vi "UPRcontroller_v00_basedonlsmv66.vi"() -> ()   [LabVIEW 2015] (continued)
                    n2964 = local read "square matrix"() -> (w6486:bool)
                    n2965 = local read "Vx-max ref"() -> (w6492:dbl)
                    n2966 = local read "Vx-min ref"() -> (w6491:dbl)
                    n2967 = local read "Vy-min ref"() -> (w6488:dbl)
                    n2968 = local read "ypixels ref"() -> (w6490:i32)
                    n2969 = local read "Vy-max ref"() -> (w6489:dbl)
                    n2970 = local read "xpixels ref"() -> (w6493:i32)
                    n2971 = local read "Angle ref"() -> (w6485:dbl)
                    n2972 = local read "Colormap"() -> (w6494:i32)
                    n2973 = call "2pparameters.vi"("command"="get") -> ("params out"=w6497:T12)  [unwired: 1 in]
                    n2974 = Bundle By Name(cluster=w6497, "Xpixels Img"=w6493, "Vx-min Img"=w6491, "VX-max Img"=w6492, "Ypixels Img"=w6490, "Vy-min Img"=w6488, "Vy-max Img"=w6489, "Colormap"=w6494, "square pixels"=w6487, "square matrix"=w6486, "Angle Img"=w6485) -> (w6496:T12)
                    n2975 = call "2pparameters.vi"("Params in"=w6496, "command"="set") -> ()  [unwired: 1 out]
                    n2976 = local read "Vx-max draw"() -> (w6477:dbl)
                    n2977 = local read "Angle drawing"() -> (w6484:dbl)
                    n2978 = local read "Vx-min draw"() -> (w6478:dbl)
                    n2979 = local read "Vy-min draw"() -> (w6481:dbl)
                    n2980 = local read "ypixels draw"() -> (w6479:dbl)
                    n2981 = local read "Vy-max draw"() -> (w6480:dbl)
                    n2982 = local read "Square pixels"() -> (w6482:bool)
                    n2983 = local read "square matrix"() -> (w6483:bool)
                    n2984 = local read "xpixels draw"() -> (w6476:dbl)
                    n2985 = local read "Colormap"() -> (w6475:i32)
                    n2986 = call "2pparameters.vi"("command"="get") -> ("params out"=w6472:T12)  [unwired: 1 in]
                    n2987 = Bundle By Name(cluster=w6472, "Xpixels"=w6476, "Vxminref"=w6478, "Vxmaxref"=w6477, "Ypixels"=w6479, "Vyminref"=w6481, "Vymaxref"=w6480, "Colormap"=w6475, "square pixels"=w6482, "square matrix"=w6483, "Angle draw"=w6484) -> (w6473:T12)
                    n2988 = call "2pparameters.vi"("Params in"=w6473, "command"="set") -> ()  [unwired: 1 out]
                  }
                  frame #1 {
                    n2989 = Current VI's Path() -> (path=w6508:path)
                    n2990 = Strip Path(path=w6508) -> (stripped path=w6509:path)  [unwired: 1 out]
                    n2991 = Build Path(base path=w6509, name or relative path="subVIs\\Image\\SetROI_v4.vi") -> (appended path=w6507:path)
                    n2992 = call <vilib>:"Set Busy.vi"() -> ("error out"=w6505:errorcluster)  [unwired: 10 in, 1 out]
                    n2993 = Open VI Reference(type specifier VI Refnum (for type only)=refnum<vi> refnum, vi path=w6507, error in (no error)=w6505) -> (vi reference=w6503:refnum<vi>, error out=w6501:errorcluster)  [unwired: 3 in]
                    n2994 = call-by-ref "?"(reference=w6503, error in=w6501) -> (reference out=w6502:refnum<vi>, error out=w6500:errorcluster)  [unwired: 1 in]
                    n2995 = Close Reference(reference=w6502, error in (no error)=w6500) -> (error out=w6504:errorcluster)
                    n2996 = call <vilib>:"Unset Busy.vi"("error in (no error)"=w6504) -> ()  [unwired: 10 in, 1 out]
                    n2997 = local write "status"(w6504) -> ()
                  }
                  frame #2 {
                    n2998 = call "2pparameters.vi"("command"="get") -> ("params out"=w6534:T12)  [unwired: 1 in]
                    n2999 = Unbundle By Name(w6534) -> ("Xpixels Img"=w6533:i32, "Vx-min Img"=w6532:dbl, "VX-max Img"=w6531:dbl, "Ypixels Img"=w6530:i32, "Vy-min Img"=w6529:dbl, "Vy-max Img"=w6528:dbl, "Colormap"=w6527:u16, "square pixels"=w6526:bool, "square matrix"=w6525:bool, "Angle Img"=w6524:dbl, "Drawing Mode"=w6523:u16)
                    n3000 = local write "xpixels ref"(w6533) -> ()
                    n3001 = local write "Vx-min ref"(w6532) -> ()
                    n3002 = local write "Vx-max ref"(w6531) -> ()
                    n3003 = local write "ypixels ref"(w6530) -> ()
                    n3004 = local write "Vy-min ref"(w6529) -> ()
                    n3005 = local write "Vy-max ref"(w6528) -> ()
                    n3006 = local write "Colormap"(w6527) -> ()
                    n3007 = local write "Square pixels"(w6526) -> ()
                    n3008 = local write "square matrix"(w6525) -> ()
                    n3009 = local write "Angle ref"(w6524) -> ()
                    n3010 = local write "ROI Type"(w6523) -> ()
                    n3011 = call "2pparameters.vi"("command"="get") -> ("params out"=w6517:T12)  [unwired: 1 in]
                    n3012 = Unbundle By Name(w6517) -> ("Xpixels"=w6511:i32, "Vxminref"=w6515:dbl, "Vxmaxref"=w6514:dbl, "Ypixels"=w6510:i32, "Vyminref"=w6513:dbl, "Vymaxref"=w6512:dbl, "Colormap"=w6518:u16, "square pixels"=w6519:bool, "square matrix"=w6520:bool, "Angle draw"=w6521:dbl, "Drawing Mode"=w6522:u16)
                    n3013 = local write "Vy-max draw"(w6512) -> ()
                    n3014 = local write "Angle drawing"(w6521) -> ()
                    n3015 = local write "Colormap"(w6518) -> ()
                    n3016 = local write "Square pixels"(w6519) -> ()
                    n3017 = local write "square matrix"(w6520) -> ()
                    n3018 = local write "ROI Type"(w6522) -> ()
                    n3019 = local write "xpixels draw"(w6511) -> ()
                    n3020 = local write "ypixels draw"(w6510) -> ()
                    n3021 = local write "Vx-min draw"(w6515) -> ()
                    n3022 = local write "Vx-max draw"(w6514) -> ()
                    n3023 = local write "Vy-min draw"(w6513) -> ()
                  }
                  frame #3 {
                    n3024 = property on="ROI" class="Bool (strict)"("Val(Sgnl)"=FALSE ("x/y scan")) -> ()  [unwired: 2 in, 2 out]
                  }
                }
              }
            }
          }
          event "Xdattype": Value Change {
            n3025 = event-data() -> ()  [unwired: 1 in, 1 out]
            n3026 = case shown="True" "Xdattype" {
              frame False {
              }
              frame True {
                n3027 = stacked-sequence {
                  frame #0 {
                    n3028 = Current VI's Path() -> (path=w6547:path)
                    n3029 = Strip Path(path=w6547) -> (stripped path=w6548:path)  [unwired: 1 out]
                    n3030 = Build Path(base path=w6548, name or relative path="subVIs\\Misc\\Changedataconfig.vi") -> (appended path=w6546:path)
                    n3031 = call <vilib>:"Set Busy.vi"() -> ("error out"=w6544:errorcluster)  [unwired: 10 in, 1 out]
                    n3032 = Open VI Reference(type specifier VI Refnum (for type only)=refnum<vi> refnum, vi path=w6546, error in (no error)=w6544) -> (vi reference=w6539:refnum<vi>, error out=w6541:errorcluster)  [unwired: 3 in]
                    n3033 = call-by-ref "?"(reference=w6539, error in=w6541) -> (reference out=w6543:refnum<vi>, error out=w6542:errorcluster)  [unwired: 12 in]
                    n3034 = Close Reference(reference=w6543, error in (no error)=w6542) -> (error out=w6538:errorcluster)
                    "status" <- w6538
                    n3035 = call <vilib>:"Unset Busy.vi"("error in (no error)"=w6538) -> ()  [unwired: 10 in, 1 out]
                  }
                  frame #1 {
                    n3036 = property on="Xdattype" class="Bool (strict)"("Val(Sgnl)"=FALSE ("x/y scan")) -> ()  [unwired: 2 in, 2 out]
                  }
                }
              }
            }
          }
          event "XautoOD": Value Change {
            n3037 = event-data() -> ()  [unwired: 1 in, 1 out]
            n3038 = case shown="True" "XautoOD" {
              frame False {
              }
              frame True {
                n3039 = stacked-sequence {
                  frame #0 {
                    n3040 = Current VI's Path() -> (path=w6560:path)
                    n3041 = Strip Path(path=w6560) -> (stripped path=w6561:path)  [unwired: 1 out]
                    n3042 = Build Path(base path=w6561, name or relative path="subVIs\\Misc\\ChangeautoODs.vi") -> (appended path=w6559:path)
                    n3043 = call <vilib>:"Set Busy.vi"() -> ("error out"=w6557:errorcluster)  [unwired: 10 in, 1 out]
                    n3044 = Open VI Reference(type specifier VI Refnum (for type only)=refnum<vi> refnum, vi path=w6559, error in (no error)=w6557) -> (vi reference=w6552:refnum<vi>, error out=w6554:errorcluster)  [unwired: 3 in]
                    n3045 = call-by-ref "?"(reference=w6552, error in=w6554) -> (reference out=w6556:refnum<vi>, error out=w6555:errorcluster)  [unwired: 12 in]
                    n3046 = Close Reference(reference=w6556, error in (no error)=w6555) -> (error out=w6551:errorcluster)
                    "status 2" <- w6551
                    n3047 = call <vilib>:"Unset Busy.vi"("error in (no error)"=w6551) -> ()  [unwired: 10 in, 1 out]
                  }
                  frame #1 {
                    n3048 = property on="XautoOD" class="Bool (strict)"("Val(Sgnl)"=FALSE ("x/y scan")) -> ()  [unwired: 2 in, 2 out]
                  }
                }
              }
            }
          }
          event "SetMan": Value Change {
            n3049 = event-data() -> ()  [unwired: 1 in, 1 out]
            n3050 = case shown="True" "SetMan" {
              frame False {
              }
              frame True {
                n3051 = stacked-sequence {
                  frame #0 {
                    w6564 = u16 0 items=["Rectangle", "Circle", "Freeform Boundary", "Freeform Interior"] ("ROI Type")
                    n3052 = local write "ROI Type"(w6564) -> ()
                    n3053 = local read "Square pixels"() -> (w6570:bool)
                    n3054 = case shown="False" w6570 {
                      frame False {
                        n3055 = local read "square matrix"() -> (w6571:bool)
                        n3056 = case shown="False" w6571 {
                          frame False {
                            "ypixels ref" <- "ypixels"
                            "xpixels ref" <- "xpixels"
                          }
                          frame True {
                            n3057 = local read "xpixels"() -> (w6576:i32)
                            n3058 = local read "ypixels"() -> (w6575:i32)
                            n3059 = Max & Min(x=w6576, y=w6575) -> (max(x,y)=w6574:i32)  [unwired: 1 out]
                            n3060 = local write "xpixels ref"(w6574) -> ()
                            n3061 = local write "ypixels ref"(w6574) -> ()
                          }
                        }
                      }
                      frame True {
                        n3062 = local read "square matrix"() -> (w6577:bool)
                        n3063 = case shown="True" w6577 {
                          frame False {
                            n3064 = local read "Vxmax"() -> (w6591:dbl)
                            n3065 = local read "Vx-min"() -> (w6590:dbl)
                            n3066 = local read "Vy-max"() -> (w6586:dbl)
                            n3067 = local read "Vy-min"() -> (w6587:dbl)
                            n3068 = Subtract(x=w6586, y=w6587) -> (x-y=w6588:dbl)
                            n3069 = Subtract(x=w6591, y=w6590) -> (x-y=w6589:dbl)
                            n3070 = Absolute Value(x=w6588) -> (abs(x)=w6579:dbl)
                            n3071 = Absolute Value(x=w6589) -> (abs(x)=w6580:dbl)
                            n3072 = Divide(x=w6580, y=w6579) -> (x/y=w6585:dbl)
                            n3073 = Greater Or Equal?(x=w6580, y=w6579) -> (x >= y?=w6578:bool)
                            n3074 = local read "xpixels"() -> (w6584:i32)
                            n3075 = local read "ypixels"() -> (w6581:i32)
                            n3076 = case shown="False" w6578 {
                              tunnel: w6585 -> [w6596 w6599]
                              tunnel: w6584 -> [w6593 _]
                              tunnel: [w6593 w6598] -> w6583
                              tunnel: [w6592 w6597] -> w6582
                              tunnel: w6581 -> [_ w6597]
                              frame False {
                                n3077 = To Double Precision Float(number=w6593) -> (double precision float=w6595:dbl)
                                n3078 = Divide(x=w6595, y=w6596) -> (x/y=w6594:dbl)
                                n3079 = To Long Integer(number=w6594) -> (32bit integer=w6592:i32)
                              }
                              frame True {
                                n3080 = To Double Precision Float(number=w6597) -> (double precision float=w6601:dbl)
                                n3081 = Multiply(x=w6601, y=w6599) -> (x*y=w6600:dbl)
                                n3082 = To Long Integer(number=w6600) -> (32bit integer=w6598:i32)
                              }
                            }
                            n3083 = local write "ypixels ref"(w6582) -> ()
                            n3084 = local write "xpixels ref"(w6583) -> ()
                          }
                          frame True {
                          }
                        }
                      }
                    }
                    "Vx-max ref" <- "Vxmax"
                    "Vx-min ref" <- "Vx-min"
                    "Vy-max ref" <- "Vy-max"
                    "Vy-min ref" <- "Vy-min"
                    "Angle ref" <- "Angle"
                  }
                  frame #1 {
                    n3085 = property on="SetMan" class="Bool (strict)"("Val(Sgnl)"=FALSE ("Value (Signaling)")) -> ()  [unwired: 2 in, 2 out]
                  }
                }
              }
            }
          }
          event "QuickSetMan": Value Change {
            n3086 = event-data() -> ()  [unwired: 1 in, 6 out]
            n3087 = case shown="True" "QuickSetMan" {
              tunnel: "Vpp" -> [_ w6607]
              tunnel: "px" -> [_ w6606]
              frame False {
              }
              frame True {
                n3088 = stacked-sequence {
                  tunnel: w6607 -> [w6612 _]
                  tunnel: w6606 -> [w6608 _]
                  frame #0 {
                    w6614 = u16 0 items=["Rectangle", "Circle", "Freeform Boundary", "Freeform Interior"] ("ROI Type")
                    n3089 = Divide(x=w6612, y=2.0) -> (x/y=w6611:dbl)
                    n3090 = Negate(x=w6611) -> (-x=w6610:dbl)
                    n3091 = local write "ROI Type"(w6614) -> ()
                    n3092 = local write "Vx-min ref"(w6610) -> ()
                    n3093 = local write "Vy-max ref"(w6611) -> ()
                    n3094 = local write "Vx-max ref"(w6611) -> ()
                    n3095 = local write "Vy-min ref"(w6610) -> ()
                    n3096 = local write "Angle ref"(0.0 ("Angle ref 2")) -> ()
                    n3097 = local write "xpixels ref"(w6608) -> ()
                    n3098 = local write "ypixels ref"(w6608) -> ()
                  }
                  frame #1 {
                    n3099 = property on="QuickSetMan" class="Bool (strict)"("Val(Sgnl)"=FALSE ("Value (Signaling)")) -> ()  [unwired: 2 in, 2 out]
                  }
                }
              }
            }
          }
          event "SetMan 2": Value Change {
            n3100 = event-data() -> ()  [unwired: 1 in, 1 out]
            n3101 = case shown="True" "SetMan 2" {
              frame False {
              }
              frame True {
                n3102 = stacked-sequence {
                  frame #0 {
                    n3103 = local write "Vx-ref"("Vx") -> ()
                    n3104 = local write "Vy-ref"("Vy") -> ()
                  }
                  frame #1 {
                    n3105 = property on="SetMan 2" class="Bool (strict)"("Val(Sgnl)"=FALSE ("Value (Signaling)")) -> ()  [unwired: 2 in, 2 out]
                  }
                }
              }
            }
          }
          event "Reset Coords": Value Change {
            n3106 = event-data() -> ("NewVal"=w6620:bool)  [unwired: 1 in, 5 out]
            n3107 = case shown="True" w6620 {
              frame False {
              }
              frame True {
                n3108 = stacked-sequence {
                  frame #0 {
                    n3109 = local write "xpixels"(256 ("xpixels")) -> ()
                    n3110 = local write "ypixels"(256 ("ypixels")) -> ()
                    n3111 = local write "Vxmax"(9.0 ("Vx-max")) -> ()
                    n3112 = local write "Vx-min"(-9.0 ("Vx-min")) -> ()
                    n3113 = local write "Vy-max"(9.0 ("Vy-max")) -> ()
                    n3114 = local write "Vy-min"(-9.0 ("Vy-min")) -> ()
                    n3115 = local write "Angle"(0.0 ("Angle")) -> ()
                  }
                  frame #1 {
                    n3116 = property on="Reset Coords" class="Bool (strict)"("Value"=FALSE ("TROI")) -> ()  [unwired: 2 in, 2 out]
                  }
                }
              }
            }
          }
          event "TROI": Value Change {
            n3117 = event-data() -> ()  [unwired: 1 in, 1 out]
            n3118 = case shown="True" "TROI" {
              frame False {
              }
              frame True {
                n3119 = stacked-sequence {
                  frame #0 {
                    n3120 = local read "Vy-min ref"() -> (w6634:dbl)
                    n3121 = local read "Vy-max ref"() -> (w6633:dbl)
                    n3122 = local read "Vx-max ref"() -> (w6631:dbl)
                    n3123 = local read "Vx-min ref"() -> (w6632:dbl)
                    n3124 = local read "ypixels ref"() -> (w6636:i32)
                    n3125 = local read "xpixels ref"() -> (w6635:i32)
                    n3126 = local read "Angle ref"() -> (w6630:dbl)
                    n3127 = local write "Angle"(w6630) -> ()
                    n3128 = local write "xpixels"(w6635) -> ()
                    n3129 = local write "Vy-min"(w6634) -> ()
                    n3130 = local write "Vy-max"(w6633) -> ()
                    n3131 = local write "Vx-min"(w6632) -> ()
                    n3132 = local write "ypixels"(w6636) -> ()
                    n3133 = local write "Vxmax"(w6631) -> ()
                  }
                  frame #1 {
                    n3134 = property on="TROI" class="Bool (strict)"("Value"=FALSE ("TROI")) -> ()  [unwired: 2 in, 2 out]
                  }
                }
              }
            }
          }
          event "TROI 2": Value Change {
            n3135 = event-data() -> ()  [unwired: 1 in, 1 out]
            n3136 = case shown="True" "TROI 2" {
              frame False {
              }
              frame True {
                n3137 = stacked-sequence {
                  frame #0 {
                    n3138 = local read "Vx-ref"() -> (w6639:dbl)
                    n3139 = local read "Vy-ref"() -> (w6640:dbl)
                    n3140 = local write "Vx"(w6639) -> ()
                    n3141 = local write "Vy"(w6640) -> ()
                  }
                  frame #1 {
                    n3142 = property on="TROI 2" class="Bool (strict)"("Value"=FALSE ("TROI")) -> ()  [unwired: 2 in, 2 out]
                  }
                }
              }
            }
          }
          event "Square pixels": Value Change {
            n3143 = event-data() -> ()  [unwired: 1 in, 1 out]
            n3144 = case shown="True" "Square pixels" {
              frame False {
              }
              frame True {
                n3145 = property on="square matrix" class="Bool (strict)"("Value"=FALSE ("square matrix")) -> ()  [unwired: 2 in, 2 out]
                n3146 = property on="Square pixels" class="Bool (strict)"("Value"=TRUE ("square matrix")) -> ()  [unwired: 2 in, 2 out]
              }
            }
          }
          event "square matrix": Value Change {
            n3147 = event-data() -> ()  [unwired: 1 in, 1 out]
            n3148 = case shown="True" "square matrix" {
              frame False {
              }
              frame True {
                n3149 = property on="square matrix" class="Bool (strict)"("Value"=TRUE ("square matrix")) -> ()  [unwired: 2 in, 2 out]
                n3150 = property on="Square pixels" class="Bool (strict)"("Value"=FALSE ("square matrix")) -> ()  [unwired: 2 in, 2 out]
              }
            }
          }
          event "up", "downright", "down", "downleft", "right", "left", "upright", "upleft": Value Change {
            n3151 = event-data() -> ()  [unwired: 1 in, 6 out]
            n3152 = local read "downright"() -> (w6653:bool)
            n3153 = local read "downleft"() -> (w6655:bool)
            n3154 = local read "upright"() -> (w6651:bool)
            n3155 = local read "upleft"() -> (w6649:bool)
            n3156 = local read "down"() -> (w6654:bool)
            n3157 = local read "right"() -> (w6652:bool)
            n3158 = local read "left"() -> (w6656:bool)
            n3159 = local read "up"() -> (w6650:bool)
            n3160 = Compound Arithmetic op=OR(w6649, w6650, w6651, w6652, w6653, w6654, w6655, w6656) -> (w6648:bool)
            n3161 = case shown="True" w6648 {
              frame False {
              }
              frame True {
                n3162 = stacked-sequence {
                  frame #0 {
                    n3163 = local read "downright"() -> (w6658:bool)
                    n3164 = local read "downleft"() -> (w6660:bool)
                    n3165 = local read "BigSmall"() -> (w6657:bool)
                    n3166 = local read "upright"() -> (w6662:bool)
                    n3167 = local read "upleft"() -> (w6665:bool)
                    n3168 = local read "down"() -> (w6661:bool)
                    n3169 = local read "right"() -> (w6663:bool)
                    n3170 = local read "left"() -> (w6659:bool)
                    n3171 = local read "up"() -> (w6664:bool)
                    n3172 = call "movestageparams.vi"("command"="get") -> ("Params out"=w6668:T23)  [unwired: 1 in]
                    n3173 = Bundle By Name(cluster=w6668, "upleft"=w6665, "up"=w6664, "upright"=w6662, "right"=w6663, "downright"=w6658, "down"=w6661, "downleft"=w6660, "left"=w6659, "Bigsmall"=w6657) -> (w6669:T23)
                    n3174 = call "movestageparams.vi"("Params in"=w6669, "command"="set") -> ()  [unwired: 1 out]
                  }
                  frame #1 {
                    n3175 = disable-structure shown="Disabled" {
                      frame Disabled {
                        n3176 = call "configuration.vi"("command"="get") -> ("config out"=w6672:T14)  [unwired: 2 in, 1 out]
                        n3177 = in-place {
                          n3178 = in-place-cluster #45(w6672) -> ()  [unwired: 2 out]
                          n3179 = in-place-cluster #45("StageL"="StageL", "StageS"="StageS") -> (w6670:T14)
                        }
                        n3180 = call "configuration.vi"("config in"=w6670, "command"="set") -> ()  [unwired: 1 in, 2 out]
                      }
                      frame Enabled {
                      }
                    }
                  }
                  frame #2 {
                    n3181 = call "movestage.vi"() -> ()  [unwired: 12 in]
                  }
                  frame #3 {
                    w6676 = FALSE ("OK Button")
                    w6677 = FALSE ("OK Button")
                    n3182 = property on="down" class="Bool (strict)"("Value"=w6677) -> ()  [unwired: 2 in, 2 out]
                    n3183 = property on="up" class="Bool (strict)"("Value"=w6677) -> ()  [unwired: 2 in, 2 out]
                    n3184 = property on="right" class="Bool (strict)"("Value"=w6677) -> ()  [unwired: 2 in, 2 out]
                    n3185 = property on="left" class="Bool (strict)"("Value"=w6677) -> ()  [unwired: 2 in, 2 out]
                    n3186 = property on="upright" class="Bool (strict)"("Value"=w6676) -> ()  [unwired: 2 in, 2 out]
                    n3187 = property on="downleft" class="Bool (strict)"("Value"=w6676) -> ()  [unwired: 2 in, 2 out]
                    n3188 = property on="downright" class="Bool (strict)"("Value"=w6676) -> ()  [unwired: 2 in, 2 out]
                    n3189 = property on="upleft" class="Bool (strict)"("Value"=w6676) -> ()  [unwired: 2 in, 2 out]
                  }
                }
              }
            }
          }
          event "finite samples": Value Change {
            n3190 = event-data() -> ("NewVal"=w6678:bool)  [unwired: 1 in]
            n3191 = flat-sequence {
              tunnel: w6678 -> [w6679]
              frame #0 {
                n3192 = case shown="True" w6679 {
                  frame False {
                    w6680 = FALSE ("wavdet")
                    n3193 = property on="continuous" class="Bool (strict)"("Value"=TRUE ("continuous for display")) -> ()  [unwired: 2 in, 2 out]
                    n3194 = property on="wavdet" class="Bool (strict)"("Value"=w6680) -> ()  [unwired: 2 in, 2 out]
                    n3195 = property on="save\ndata" class="Bool (strict)"("Value"=w6680) -> ()  [unwired: 2 in, 2 out]
                    n3196 = property on="# of frames" class="DigNum (strict)"("DisabledEnum"=T8."Disabled and Grayed Out" ("Disabled")) -> ()  [unwired: 2 in, 2 out]
                    n3197 = property on="save\ndata" class="Bool (strict)"("DisabledEnum"=T8."Disabled and Grayed Out" ("Disabled")) -> ()  [unwired: 2 in, 2 out]
                    "Save tab" <- enum32{"withsave", "withoutsave"}."withsave" ("Save tab")
                  }
                  frame True {
                    w6687 = FALSE ("continuous for display")
                    n3198 = property on="continuous" class="Bool (strict)"("Value"=w6687) -> ()  [unwired: 2 in, 2 out]
                    n3199 = property on="wavdet" class="Bool (strict)"("Value"=w6687) -> ()  [unwired: 2 in, 2 out]
                    n3200 = local write "Save tab"(enum32{"withsave", "withoutsave"}."withsave" ("Save tab")) -> ()
                    n3201 = property on="save\ndata" class="Bool (strict)"("DisabledEnum"=T8."Enabled" ("Disabled")) -> ()  [unwired: 2 in, 2 out]
                    n3202 = property on="save\ndata" class="Bool (strict)"("Value"=TRUE ("save\ndata")) -> ()  [unwired: 2 in, 2 out]
                    n3203 = property on="# of frames" class="DigNum (strict)"("DisabledEnum"=T8."Enabled" ("Disabled")) -> ()  [unwired: 2 in, 2 out]
                  }
                }
              }
              frame #1 {
                n3204 = local read "finite samples"() -> (w6696:bool)
                n3205 = local read "continuous"() -> (w6695:bool)
                n3206 = local read "wavdet"() -> (w6694:bool)
                n3207 = call "2pparameters.vi"("command"="get") -> ("params out"=w6690:T12)  [unwired: 1 in]
                n3208 = Bundle By Name(cluster=w6690, "finite"=w6696, "cont"=w6695, "wavdet"=w6694) -> (w6693:T12)
                n3209 = call "2pparameters.vi"("Params in"=w6693, "command"="set") -> ()  [unwired: 1 out]
              }
            }
          }
          event "continuous": Value Change {
            n3210 = event-data() -> ("NewVal"=w6697:bool)  [unwired: 1 in]
            n3211 = flat-sequence {
              tunnel: w6697 -> [w6698]
              frame #0 {
                n3212 = case shown="True" w6698 {
                  frame False {
                    n3213 = property on="finite samples" class="Bool (strict)"("Value"=TRUE ("finite samples for recording")) -> ()  [unwired: 2 in, 2 out]
                    n3214 = property on="save\ndata" class="Bool (strict)"("Value"=TRUE ("save\ndata")) -> ()  [unwired: 2 in, 2 out]
                    n3215 = property on="wavdet" class="Bool (strict)"("Value"=FALSE ("wavdet")) -> ()  [unwired: 2 in, 2 out]
                    n3216 = local write "Save tab"(enum32{"withsave", "withoutsave"}."withsave" ("Save tab")) -> ()
                    n3217 = property on="# of frames" class="DigNum (strict)"("DisabledEnum"=T8."Enabled" ("Disabled")) -> ()  [unwired: 2 in, 2 out]
                    n3218 = property on="save\ndata" class="Bool (strict)"("DisabledEnum"=T8."Enabled" ("Disabled")) -> ()  [unwired: 2 in, 2 out]
                  }
                  frame True {
                    w6705 = FALSE ("finite samples for recording")
                    n3219 = property on="finite samples" class="Bool (strict)"("Value"=w6705) -> ()  [unwired: 2 in, 2 out]
                    n3220 = property on="wavdet" class="Bool (strict)"("Value"=w6705) -> ()  [unwired: 2 in, 2 out]
                    n3221 = property on="save\ndata" class="Bool (strict)"("Value"=w6705) -> ()  [unwired: 2 in, 2 out]
                    n3222 = local write "Save tab"(enum32{"withsave", "withoutsave"}."withsave" ("Save tab")) -> ()
                    n3223 = property on="# of frames" class="DigNum (strict)"("DisabledEnum"=T8."Disabled and Grayed Out" ("Disabled")) -> ()  [unwired: 2 in, 2 out]
                    n3224 = property on="save\ndata" class="Bool (strict)"("DisabledEnum"=T8."Disabled and Grayed Out" ("Disabled")) -> ()  [unwired: 2 in, 2 out]
                  }
                }
              }
              frame #1 {
                n3225 = local read "finite samples"() -> (w6715:bool)
                n3226 = local read "continuous"() -> (w6714:bool)
                n3227 = local read "wavdet"() -> (w6713:bool)
                n3228 = call "2pparameters.vi"("command"="get") -> ("params out"=w6709:T12)  [unwired: 1 in]
                n3229 = Bundle By Name(cluster=w6709, "finite"=w6715, "cont"=w6714, "wavdet"=w6713) -> (w6712:T12)
                n3230 = call "2pparameters.vi"("Params in"=w6712, "command"="set") -> ()  [unwired: 1 out]
              }
            }
          }
          event "wavdet": Value Change {
            n3231 = event-data() -> ("NewVal"=w6716:bool)  [unwired: 1 in]
            n3232 = flat-sequence {
              tunnel: w6716 -> [w6717]
              frame #0 {
                n3233 = case shown="False" w6717 {
                  frame False {
                    n3234 = property on="finite samples" class="Bool (strict)"("Value"=TRUE ("finite samples for recording")) -> ()  [unwired: 2 in, 2 out]
                    n3235 = property on="continuous" class="Bool (strict)"("Value"=FALSE ("continuous")) -> ()  [unwired: 2 in, 2 out]
                    n3236 = local write "Save tab"(enum32{"withsave", "withoutsave"}."withsave" ("Save tab")) -> ()
                    n3237 = property on="save\ndata" class="Bool (strict)"("DisabledEnum"=T8."Enabled" ("Disabled")) -> ()  [unwired: 2 in, 2 out]
                    n3238 = property on="# of frames" class="DigNum (strict)"("DisabledEnum"=T8."Enabled" ("Disabled")) -> ()  [unwired: 2 in, 2 out]
                    n3239 = property on="save\ndata" class="Bool (strict)"("Value"=TRUE ("save\ndata")) -> ()  [unwired: 2 in, 2 out]
                  }
                  frame True {
                    w6726 = FALSE ("finite samples for recording")
                    n3240 = property on="finite samples" class="Bool (strict)"("Value"=w6726) -> ()  [unwired: 2 in, 2 out]
                    n3241 = property on="continuous" class="Bool (strict)"("Value"=w6726) -> ()  [unwired: 2 in, 2 out]
                    n3242 = property on="save\ndata" class="Bool (strict)"("DisabledEnum"=T8."Enabled" ("Disabled")) -> ()  [unwired: 2 in, 2 out]
                    n3243 = local write "Save tab"(enum32{"withsave", "withoutsave"}."withsave" ("Save tab")) -> ()
                    n3244 = property on="# of frames" class="DigNum (strict)"("DisabledEnum"=T8."Disabled" ("Disabled")) -> ()  [unwired: 2 in, 2 out]
                    n3245 = property on="save\ndata" class="Bool (strict)"("Value"=TRUE ("save\ndata")) -> ()  [unwired: 2 in, 2 out]
                  }
                }
              }
              frame #1 {
                n3246 = local read "finite samples"() -> (w6729:bool)
                n3247 = local read "continuous"() -> (w6730:bool)
                n3248 = local read "wavdet"() -> (w6731:bool)
                n3249 = call "2pparameters.vi"("command"="get") -> ("params out"=w6735:T12)  [unwired: 1 in]
                n3250 = Bundle By Name(cluster=w6735, "finite"=w6729, "cont"=w6730, "wavdet"=w6731) -> (w6732:T12)
                n3251 = call "2pparameters.vi"("Params in"=w6732, "command"="set") -> ()  [unwired: 1 out]
              }
            }
          }
          event "cursors": Value Change {
            n3252 = event-data() -> ()  [unwired: 1 in, 5 out]
            n3253 = case shown="True" "cursors" {
              frame False {
                n3254 = property on="img_CH1" class="IntGraph (strict)"("Active Cursor"=u32 0, "Cursor.Cursor Style"=u8 0 ("Cursor Style"), "Cursor.Cursor Point Style"=u8 0 ("Cursor Point Style")) -> ("Cursor.Cursor Position:Cursor X"=w6740:dbl, "Cursor.Cursor Position:Cursor Y"=w6741:dbl)  [unwired: 2 in, 2 out]
                n3255 = property on="img_CH2" class="IntGraph (strict)"("Active Cursor"=u32 0, "Cursor.Cursor Style"=u8 0 ("Cursor Style"), "Cursor.Cursor Point Style"=u8 0 ("Cursor Point Style")) -> ()  [unwired: 2 in, 2 out]
                n3256 = local write "cursor x [pixel]"(w6740) -> ()
                n3257 = local write "cursor y [pixel]"(w6741) -> ()
              }
              frame True {
                n3258 = stacked-sequence {
                  frame #0 {
                    n3259 = call "2pparameters.vi"("command"="get") -> ("params out"=w6756:T12)  [unwired: 1 in]
                    n3260 = Unbundle By Name(w6756) -> ("Xpixels Img"=w6757:i32, "Ypixels Img"=w6754:i32)
                    n3261 = To Double Precision Float(number=w6754) -> (double precision float=w6748:dbl)
                    n3262 = To Double Precision Float(number=w6757) -> (double precision float=w6753:dbl)
                    n3263 = Divide(x=w6748, y=2.0) -> (x/y=w6749:dbl)
                    n3264 = Divide(x=w6753, y=2.0) -> (x/y=w6751:dbl)
                    n3265 = Round To Nearest(number=w6749) -> (nearest integer value=w6747:dbl)
                    n3266 = Round To Nearest(number=w6751) -> (nearest integer value=w6750:dbl)
                    n3267 = property on="img_CH1" class="IntGraph (strict)"("Active Cursor"=u32 0, "Cursor.Cursor Style"=u8 8 ("Cursor Style"), "Cursor.Cursor Point Style"=u8 5 ("Cursor Point Style"), "Cursor.Cursor Position:Cursor X"=w6750, "Cursor.Cursor Position:Cursor Y"=w6747, "Cursor.Visible"=TRUE) -> ()  [unwired: 2 in, 2 out]
                  }
                  frame #1 {
                    n3268 = call "2pparameters.vi"("command"="get") -> ("params out"=w6776:T12)  [unwired: 1 in]
                    n3269 = call "2pparameters.vi"("command"="get") -> ("params out"=w6774:T12)  [unwired: 1 in]
                    n3270 = property on="img_CH1" class="IntGraph (strict)"("Active Cursor"=u32 0, "Cursor.Cursor Style"=u8 8 ("Cursor Style"), "Cursor.Cursor Point Style"=u8 5 ("Cursor Point Style")) -> ("Cursor.Cursor Position:Cursor X"=w6769:dbl, "Cursor.Cursor Position:Cursor Y"=w6768:dbl, "Cursor.Cursor Index"=w6791:i32, "Cursor.Cursor Plot"=w6790:i32, "Cursor.Visible"=w6761:bool)  [unwired: 2 in, 2 out]
                    "cursor x [pixel]" <- w6769
                    "cursor y [pixel]" <- w6768
                    n3271 = Unbundle By Name(w6776) -> ("Vy-max Img"=w6778:dbl, "Vy-min Img"=w6765:dbl, "Ypixels Img"=w6780:i32)
                    n3272 = Unbundle By Name(w6774) -> ("VX-max Img"=w6775:dbl, "Vx-min Img"=w6763:dbl, "Xpixels Img"=w6779:i32)
                    n3273 = Subtract(x=w6778, y=w6765) -> (x-y=w6783:dbl)
                    n3274 = Subtract(x=w6775, y=w6763) -> (x-y=w6781:dbl)
                    n3275 = local read "img_CH2"() -> (w6787:sgl[][])
                    n3276 = To Double Precision Float(number=w6779) -> (double precision float=w6782:dbl)
                    n3277 = local read "img_CH1"() -> (w6788:sgl[][])
                    n3278 = To Double Precision Float(number=w6780) -> (double precision float=w6784:dbl)
                    n3279 = Index Array(array=w6788, index (row)=w6791, index (col)=w6790) -> (element=→"value CH 1":sgl)
                    n3280 = Index Array(array=w6787, index (row)=w6791, index (col)=w6790) -> (element=→"value CH 2":sgl)
                    n3281 = Divide(x=w6781, y=w6782) -> (x/y=w6785:dbl)
                    n3282 = Divide(x=w6783, y=w6784) -> (x/y=w6786:dbl)
                    n3283 = Multiply(x=w6769, y=w6785) -> (x*y=w6764:dbl)
                    n3284 = Multiply(x=w6768, y=w6786) -> (x*y=w6767:dbl)
                    n3285 = property on="img_CH2" class="IntGraph (strict)"("Active Cursor"=u32 0, "Cursor.Cursor Style"=u8 8 ("Cursor Style"), "Cursor.Cursor Point Style"=u8 5 ("Cursor Point Style"), "Cursor.Cursor Position:Cursor X"=w6769, "Cursor.Cursor Position:Cursor Y"=w6768, "Cursor.Visible"=w6761) -> ()  [unwired: 2 in, 2 out]
                    n3286 = Add(x=w6764, y=w6763) -> (x+y=w6762:dbl)
                    n3287 = Add(x=w6767, y=w6765) -> (x+y=w6766:dbl)
                    n3288 = local write "Vx-ref"(w6762) -> ()
                    n3289 = local write "Vy-ref"(w6766) -> ()
                  }
                }
              }
            }
          }
          event "img_CH1": Cursor Move {
            n3290 = event-data() -> ("CursIdx"=w6796:i32)  [unwired: 1 in]
            n3291 = Equal To 0?(x=w6796) -> (x = 0?=w6797:bool)
            n3292 = case shown="True" w6797 {
              frame False {
              }
              frame True {
                n3293 = call "2pparameters.vi"("command"="get") -> ("params out"=w6817:T12)  [unwired: 1 in]
                n3294 = call "2pparameters.vi"("command"="get") -> ("params out"=w6819:T12)  [unwired: 1 in]
                n3295 = property on="img_CH1" class="IntGraph (strict)"("Active Cursor"=u32 0, "Cursor.Cursor Style"=u8 8 ("Cursor Style"), "Cursor.Cursor Point Style"=u8 5 ("Cursor Point Style")) -> ("Cursor.Cursor Position:Cursor X"=w6806:dbl, "Cursor.Cursor Position:Cursor Y"=w6805:dbl, "Cursor.Cursor Plot"=w6825:i32, "Cursor.Cursor Index"=w6824:i32, "Cursor.Visible"=w6798:bool)  [unwired: 2 in, 2 out]
                n3296 = Unbundle By Name(w6817) -> ("Vy-max Img"=w6815:dbl, "Vy-min Img"=w6804:dbl, "Ypixels Img"=w6813:i32)
                n3297 = Unbundle By Name(w6819) -> ("VX-max Img"=w6818:dbl, "Vx-min Img"=w6799:dbl, "Xpixels Img"=w6814:i32)
                n3298 = Subtract(x=w6815, y=w6804) -> (x-y=w6810:dbl)
                n3299 = Subtract(x=w6818, y=w6799) -> (x-y=w6812:dbl)
                n3300 = local write "cursor x [pixel]"(w6806) -> ()
                n3301 = local write "cursor y [pixel]"(w6805) -> ()
                n3302 = To Double Precision Float(number=w6814) -> (double precision float=w6811:dbl)
                n3303 = To Double Precision Float(number=w6813) -> (double precision float=w6809:dbl)
                n3304 = local read "img_CH2"() -> (w6826:sgl[][])
                n3305 = local read "img_CH1"() -> (w6829:sgl[][])
                n3306 = Index Array(array=w6826, index (row)=w6825, index (col)=w6824) -> (element=w6827:sgl)
                n3307 = Index Array(array=w6829, index (row)=w6825, index (col)=w6824) -> (element=w6828:sgl)
                n3308 = Divide(x=w6812, y=w6811) -> (x/y=w6808:dbl)
                n3309 = Divide(x=w6810, y=w6809) -> (x/y=w6807:dbl)
                n3310 = local write "value CH 2"(w6827) -> ()
                n3311 = Multiply(x=w6806, y=w6808) -> (x*y=w6801:dbl)
                n3312 = local write "value CH 1"(w6828) -> ()
                n3313 = Multiply(x=w6805, y=w6807) -> (x*y=w6803:dbl)
                n3314 = Add(x=w6801, y=w6799) -> (x+y=w6800:dbl)
                n3315 = local write "Vx-ref"(w6800) -> ()
                n3316 = Add(x=w6803, y=w6804) -> (x+y=w6802:dbl)
                n3317 = property on="img_CH2" class="IntGraph (strict)"("Active Cursor"=u32 0, "Cursor.Cursor Style"=u8 8 ("Cursor Style"), "Cursor.Cursor Point Style"=u8 5 ("Cursor Point Style"), "Cursor.Cursor Position:Cursor X"=w6806, "Cursor.Cursor Position:Cursor Y"=w6805, "Cursor.Visible"=w6798) -> ()  [unwired: 2 in, 2 out]
                n3318 = local write "Vy-ref"(w6802) -> ()
              }
            }
          }
          event "img_CH2": Cursor Move {
            n3319 = event-data() -> ("CursIdx"=w6833:i32)  [unwired: 1 in]
            n3320 = Equal To 0?(x=w6833) -> (x = 0?=w6834:bool)
            n3321 = case shown="True" w6834 {
              frame False {
              }
              frame True {
                n3322 = property on="img_CH2" class="IntGraph (strict)"("Active Cursor"=u32 0, "Cursor.Cursor Style"=u8 8 ("Cursor Style"), "Cursor.Cursor Point Style"=u8 5 ("Cursor Point Style")) -> ("Cursor.Cursor Position:Cursor X"=w6842:dbl, "Cursor.Cursor Position:Cursor Y"=w6843:dbl, "Cursor.Cursor Plot"=w6862:i32, "Cursor.Cursor Index"=w6861:i32, "Cursor.Visible"=w6835:bool)  [unwired: 2 in, 2 out]
                n3323 = call "2pparameters.vi"("command"="get") -> ("params out"=w6854:T12)  [unwired: 1 in]
                n3324 = call "2pparameters.vi"("command"="get") -> ("params out"=w6856:T12)  [unwired: 1 in]
                n3325 = local read "img_CH1"() -> (w6866:sgl[][])
                n3326 = local read "img_CH2"() -> (w6863:sgl[][])
                n3327 = local write "cursor x [pixel]"(w6842) -> ()
                n3328 = local write "cursor y [pixel]"(w6843) -> ()
                n3329 = Unbundle By Name(w6854) -> ("Vy-max Img"=w6852:dbl, "Vy-min Img"=w6837:dbl, "Ypixels Img"=w6850:i32)
                n3330 = Unbundle By Name(w6856) -> ("VX-max Img"=w6855:dbl, "Vx-min Img"=w6840:dbl, "Xpixels Img"=w6851:i32)
                n3331 = Index Array(array=w6866, index (row)=w6862, index (col)=w6861) -> (element=w6865:sgl)
                n3332 = Index Array(array=w6863, index (row)=w6862, index (col)=w6861) -> (element=w6864:sgl)
                n3333 = local write "value CH 2"(w6864) -> ()
                n3334 = local write "value CH 1"(w6865) -> ()
                n3335 = Subtract(x=w6852, y=w6837) -> (x-y=w6847:dbl)
                n3336 = Subtract(x=w6855, y=w6840) -> (x-y=w6849:dbl)
                n3337 = To Double Precision Float(number=w6851) -> (double precision float=w6848:dbl)
                n3338 = To Double Precision Float(number=w6850) -> (double precision float=w6846:dbl)
                n3339 = Divide(x=w6849, y=w6848) -> (x/y=w6845:dbl)
                n3340 = Divide(x=w6847, y=w6846) -> (x/y=w6844:dbl)
                n3341 = Multiply(x=w6842, y=w6845) -> (x*y=w6841:dbl)
                n3342 = Multiply(x=w6843, y=w6844) -> (x*y=w6838:dbl)
                n3343 = property on="img_CH1" class="IntGraph (strict)"("Active Cursor"=u32 0, "Cursor.Cursor Style"=u8 8 ("Cursor Style"), "Cursor.Cursor Point Style"=u8 5 ("Cursor Point Style"), "Cursor.Cursor Position:Cursor X"=w6842, "Cursor.Cursor Position:Cursor Y"=w6843, "Cursor.Visible"=w6835) -> ()  [unwired: 2 in, 2 out]
                n3344 = Add(x=w6841, y=w6840) -> (x+y=→"Vx-ref":dbl)
                n3345 = Add(x=w6838, y=w6837) -> (x+y=→"Vy-ref":dbl)
              }
            }
          }
          event "Focus": Value Change {
            n3346 = event-data() -> ()  [unwired: 1 in, 6 out]
            n3347 = flat-sequence {
              frame #0 {
                n3348 = local read "Focus"() -> (w6870:bool)
                n3349 = case shown="True" w6870 {
                  frame False {
                  }
                  frame True {
                    n3350 = local read "Vx-ref"() -> (w6874:dbl)
                    n3351 = local read "Vy-ref"() -> (w6873:dbl)
                    n3352 = local read "zV"() -> (w6871:dbl)
                    n3353 = call "focusvi.vi"("zc"=w6871, "yc"=w6873, "xc"=w6874) -> ("finalz"=→"zV":dbl)
                  }
                }
              }
              frame #1 {
                n3354 = local write "Focus"(FALSE ("Focus")) -> ()
              }
            }
          }
          event "auto shutter": Value Change {
            n3355 = event-data() -> ()  [unwired: 1 in, 6 out]
            n3356 = call "2pparameters.vi"("command"="get") -> ("params out"=w6878:T12)  [unwired: 1 in]
            n3357 = in-place {
              n3358 = in-place-cluster #46(w6878) -> ()  [unwired: 1 out]
              n3359 = local read "auto shutter"() -> (w6880:bool)
              n3360 = in-place-cluster #46("autoshutter"=w6880) -> (w6876:T12)
            }
            n3361 = call "2pparameters.vi"("Params in"=w6876, "command"="set") -> ()  [unwired: 1 out]
          }
          event "auto OD": Value Change {
            n3362 = event-data() -> ()  [unwired: 1 in, 6 out]
            n3363 = call "2pparameters.vi"("command"="get") -> ("params out"=w6883:T12)  [unwired: 1 in]
            n3364 = in-place {
              n3365 = in-place-cluster #47(w6883) -> ()  [unwired: 1 out]
              n3366 = local read "auto OD"() -> (w6885:bool)
              n3367 = in-place-cluster #47("auto OD"=w6885) -> (w6881:T12)
            }
            n3368 = call "2pparameters.vi"("Params in"=w6881, "command"="set") -> ()  [unwired: 1 out]
          }
          event "ODfilt": Value Change {
            n3369 = event-data() -> ("OldVal"=w6888:u16)  [unwired: 1 in, 5 out]
            n3370 = call "2pparameters.vi"("command"="get") -> ("params out"=w6886:T12)  [unwired: 1 in]
            n3371 = local read "ODfilt"() -> (w6889:u16)
            n3372 = call "filterwheelcontrol_nothorlabslib.vi"("Current OD filt"=w6888, "New ODfilt"=w6889) -> ()  [unwired: 1 in]
            n3373 = in-place {
              in-place-border: w6889 -> [w6892]
              n3374 = in-place-cluster #48(w6886) -> ()  [unwired: 1 out]
              n3375 = in-place-cluster #48("ODfilt"=w6892) -> (w6890:T12)
            }
            n3376 = call "2pparameters.vi"("Params in"=w6890, "command"="set") -> ()  [unwired: 1 out]
          }
          event "Use external 100KHz Clock": Value Change {
            n3377 = event-data() -> ("NewVal"=w6894:bool)  [unwired: 1 in, 5 out]
            n3378 = control-ref of="Measurement"() -> (w6896:refnum<vi>)
            n3379 = property class="Enum (strict)"(reference=w6896) -> ("Value"=w6895:T4)  [unwired: 1 in, 2 out]
            n3380 = case shown="\"Timetrace\"" w6895 {
              tunnel: [w6912 w6913] -> w6893
              frame "X-Y-t movie", "X-Y-Z stack", Default {
                n3381 = control-ref of="Sampling rate"() -> (w6912:refnum<vi>)
              }
              frame "Timetrace" {
                n3382 = control-ref of="srateAODOtt"() -> (w6913:refnum<vi>)
              }
            }
            n3383 = case shown="False" w6894 {
              tunnel: w6893 -> [w6897 w6904]
              frame False {
                n3384 = call "2pparameters.vi"("command"="get") -> ("params out"=w6901:T12)  [unwired: 1 in]
                n3385 = Bundle By Name(cluster=w6901, "External 100KHz Clock?"=FALSE) -> (w6898:T12)
                n3386 = property class="DigNum (strict)"(reference=w6897, "DisabledEnum"=T8."Enabled" ("Disabled")) -> ()  [unwired: 1 in, 2 out]
                n3387 = call "2pparameters.vi"("Params in"=w6898, "command"="set") -> ()  [unwired: 1 out]
              }
              frame True {
                n3388 = property class="DigNum (strict)"(reference=w6904, "Val(Sgnl)"=100000.0 ("Value (Signaling)"), "DisabledEnum"=T8."Disabled and Grayed Out" ("Disabled")) -> ()  [unwired: 1 in, 2 out]
                n3389 = call "2pparameters.vi"("command"="get") -> ("params out"=w6910:T12)  [unwired: 1 in]
                n3390 = Bundle By Name(cluster=w6910, "External 100KHz Clock?"=TRUE) -> (w6907:T12)
                n3391 = call "2pparameters.vi"("Params in"=w6907, "command"="set") -> ()  [unwired: 1 out]
              }
            }
          }
          event "Exit": Value Change {
            n3392 = event-data() -> ()  [unwired: 1 in, 5 out]
            n3393 = disable-structure shown="Enabled" {
              frame Disabled {
                # "added to see if it would fix crasing on exit"
                n3394 = call "ROI-databuffer.vi"("command"=enum16{"get", "set", "clear", "append"}."clear") -> ()  [unwired: 4 in, 1 out]
              }
              frame Enabled {
              }
            }
          }
        }
        n3395 = Wait (ms)(milliseconds to wait=u32 50) -> ()  [unwired: 1 out]
      }
      n3396 = while {
        stop <- w82 stop-if-true
        # "Waveform generation"
        n3397 = event shown="[12] \"Load Matlab Waveform DO\": Value Change" {
          selector: _ -> [_ _ _ _ _ _ _ _ _ _ _ _ _ _ _ _ _ _ _ _ _ _]
          dyn-events: _ -> [_ _ _ _ _ _ _ _ _ _ _ _ _ _ _ _ _ _ _ _ _ _]
          timeout: _ -> [_ _ _ _ _ _ _ _ _ _ _ _ _ _ _ _ _ _ _ _ _ _]
          tunnel: [_ _ _ _ _ _ _ _ _ _ _ _ _ _ _ _ _ _ _ _ _ w2252] -> w82
          event Timeout {
            n3398 = event-data() -> ()  [unwired: 1 in, 3 out]
          }
          event "Add AO wave": Value Change {
            n3399 = event-data() -> ("NewVal"=w83:bool)  [unwired: 1 in, 5 out]
            n3400 = case shown="True" w83 {
              frame False {
              }
              frame True {
                n3401 = stacked-sequence {
                  seq-local: [_ _ w190 _ _ _ _ _] -> [_ _ _ w222 w233 w241 w307 w339]
                  frame #0 {
                    n3402 = local read "Measurement"() -> (w84:T4)
                    n3403 = case shown="\"Lifetime (contour)\"" w84 {
                      frame "X-Y-t movie", Default {
                        n3404 = local read "avpp"() -> (w105:i32)
                        n3405 = local read "Angle ref"() -> (w104:dbl)
                        n3406 = local read "ROI Type"() -> (w103:u16)
                        n3407 = local read "xpixels ref"() -> (w100:i32)
                        n3408 = local read "Vx-min ref"() -> (w99:dbl)
                        n3409 = local read "Vx-max ref"() -> (w98:dbl)
                        n3410 = local read "ypixels ref"() -> (w96:i32)
                        n3411 = local read "Vy-min ref"() -> (w97:dbl)
                        n3412 = local read "Vy-max ref"() -> (w93:dbl)
                        n3413 = local read "Sampling rate"() -> (w87:dbl)
                        n3414 = local read "finite samples"() -> (w88:bool)
                        n3415 = local read "continuous"() -> (w91:bool)
                        n3416 = local read "wavdet"() -> (w92:bool)
                        n3417 = local read "# of frames"() -> (w90:i32)
                        n3418 = local read "maxbufferAI"() -> (w89:i32)
                        n3419 = local read "Override AI buffer"() -> (w85:bool)
                        n3420 = call "2pparameters.vi"("command"="get") -> ("params out"=w102:T12)  [unwired: 1 in]
                        n3421 = Bundle By Name(cluster=w102, "type"="X-Y-t movie", "avpp"=w105, "Angle Img"=w104, "Xpixels Img"=w100, "Vx-min Img"=w99, "VX-max Img"=w98, "Ypixels Img"=w96, "Vy-min Img"=w97, "Vy-max Img"=w93, "srate"=w87, "srate Img"=w87, "finite"=w88, "cont"=w91, "wavdet"=w92, "measpoints"=w90, "maxbufferAI"=w89, "Drawing Mode"=w103, "Vz-reset"=0.0, "AIoverride"=w85) -> (w94:T12)
                        n3422 = call "2pparameters.vi"("Params in"=w94, "command"="set") -> ()  [unwired: 1 out]
                      }
                      frame "X-Y-Z stack" {
                        n3423 = call "2pparameters.vi"("command"="get") -> ("params out"=w109:T12)  [unwired: 1 in]
                        n3424 = Bundle By Name(cluster=w109, "type"="X-Y-Z stack") -> (w107:T12)
                        n3425 = call "2pparameters.vi"("Params in"=w107, "command"="set") -> ()  [unwired: 1 out]
                      }
                      frame "Lifetime (scan)" {
                        n3426 = call "2pparameters.vi"("command"="get") -> ("params out"=w114:T12)  [unwired: 1 in]
                        n3427 = Bundle By Name(cluster=w114, "type"="Lifetime (scan)") -> (w112:T12)
                        n3428 = call "2pparameters.vi"("Params in"=w112, "command"="set") -> ()  [unwired: 1 out]
                      }
                      frame "Lifetime (contour)" {
                        n3429 = local read "Vy-min draw"() -> (w124:dbl)
                        n3430 = local read "Vy-max draw"() -> (w123:dbl)
                        n3431 = local read "Vx-min draw"() -> (w126:dbl)
                        n3432 = local read "Vx-max draw"() -> (w125:dbl)
                        n3433 = local read "xpixels ref"() -> (w122:i32)
                        n3434 = local read "ypixels ref"() -> (w121:i32)
                        n3435 = local read "ROI Type"() -> (w120:u16)
                        n3436 = local read "srateAODOtt"() -> (w131:dbl)
                        n3437 = local read "# of frames"() -> (w136:i32)
                        n3438 = local read "refreshtime"() -> (w128:dbl)
                        n3439 = local read "Pel"() -> (w119:dbl)
                        n3440 = local read "bin"() -> (w134:dbl)
                        n3441 = local read "Override AI buffer"() -> (w117:bool)
                        n3442 = local read "finite samples"() -> (w143:bool)
                        n3443 = local read "srateAODOtt"() -> (w130:dbl)
                        n3444 = local read "srateAODOtt"() -> (w137:dbl)
                        n3445 = local read "continuous"() -> (w142:bool)
                        n3446 = local read "Angle ref"() -> (w127:dbl)
                        n3447 = local read "wavdet"() -> (w144:bool)
                        n3448 = local read "Vx-ref"() -> (w139:dbl)
                        n3449 = local read "Vy-ref"() -> (w141:dbl)
                        n3450 = local read "avpp"() -> (w140:i32)
                        n3451 = call "tt_timeandsamples.vi"("bin"=w134, "refreshtime"=w128, "srateAODOtt"=w131, "tot#ofsamples"=w136) -> ("refreshrate"=w132:dbl, "refreshbuffer"=w133:i32, "timetracecycles"=w138:i32)  [unwired: 5 in]
                        n3452 = local read "bin"() -> (w135:dbl)
                        n3453 = call "2pparameters.vi"("command"="get") -> ("params out"=w147:T12)  [unwired: 1 in]
                        n3454 = Bundle By Name(cluster=w147, "Drawing Mode"=w120, "measpoints"=w136, "tt_cycles"=w138, "refreshbuffer"=w133, "refreshrate"=w132, "Vx-ref"=w139, "Vy-ref"=w141, "srate"=w130, "finite"=w143, "cont"=w142, "wavdet"=w144, "avpp"=w140, "srateAODO"=w137, "bufferAI"=w133, "bin"=w135, "Angle Img"=w127, "Vxminref"=w126, "Vxmaxref"=w125, "Vyminref"=w124, "Vymaxref"=w123, "Xpixels Img"=w122, "Ypixels Img"=w121, "Pel"=w119, "Vz-reset"=0.0, "AIoverride"=w117, "type"="Lifetime (contour)") -> (w145:T12)
                        n3455 = Reciprocal(x=w132) -> (1/x=w129:dbl)
                        n3456 = local write "refreshtime"(w129) -> ()
                        n3457 = call "2pparameters.vi"("Params in"=w145, "command"="set") -> ()  [unwired: 1 out]
                      }
                      frame "X-Y-Z-t movie" {
                      }
                      frame "linescan" {
                      }
                      frame "Timetrace" {
                        n3458 = local read "Vy-min draw"() -> (w157:dbl)
                        n3459 = local read "Vy-max draw"() -> (w156:dbl)
                        n3460 = local read "Vx-min draw"() -> (w159:dbl)
                        n3461 = local read "Vx-max draw"() -> (w158:dbl)
                        n3462 = local read "xpixels ref"() -> (w155:i32)
                        n3463 = local read "ypixels ref"() -> (w154:i32)
                        n3464 = local read "ROI Type"() -> (w153:u16)
                        n3465 = local read "srateAODOtt"() -> (w164:dbl)
                        n3466 = local read "# of frames"() -> (w169:i32)
                        n3467 = local read "refreshtime"() -> (w161:dbl)
                        n3468 = local read "Pel"() -> (w152:dbl)
                        n3469 = local read "bin"() -> (w167:dbl)
                        n3470 = local read "Override AI buffer"() -> (w150:bool)
                        n3471 = local read "finite samples"() -> (w176:bool)
                        n3472 = local read "srateAODOtt"() -> (w163:dbl)
                        n3473 = local read "srateAODOtt"() -> (w170:dbl)
                        n3474 = local read "continuous"() -> (w175:bool)
                        n3475 = local read "Angle ref"() -> (w160:dbl)
                        n3476 = local read "wavdet"() -> (w177:bool)
                        n3477 = local read "Vx-ref"() -> (w172:dbl)
                        n3478 = local read "Vy-ref"() -> (w174:dbl)
                        n3479 = local read "avpp"() -> (w173:i32)
                        n3480 = call "tt_timeandsamples.vi"("bin"=w167, "refreshtime"=w161, "srateAODOtt"=w164, "tot#ofsamples"=w169) -> ("refreshrate"=w165:dbl, "refreshbuffer"=w166:i32, "timetracecycles"=w171:i32)  [unwired: 5 in]
                        n3481 = local read "bin"() -> (w168:dbl)
                        n3482 = call "2pparameters.vi"("command"="get") -> ("params out"=w180:T12)  [unwired: 1 in]
                        n3483 = Bundle By Name(cluster=w180, "Drawing Mode"=w153, "measpoints"=w169, "tt_cycles"=w171, "refreshbuffer"=w166, "refreshrate"=w165, "Vx-ref"=w172, "Vy-ref"=w174, "srate"=w163, "finite"=w176, "cont"=w175, "wavdet"=w177, "avpp"=w173, "srateAODO"=w170, "bufferAI"=w166, "bin"=w168, "Angle Img"=w160, "Vxminref"=w159, "Vxmaxref"=w158, "Vyminref"=w157, "Vymaxref"=w156, "Xpixels Img"=w155, "Ypixels Img"=w154, "Pel"=w152, "Vz-reset"=0.0, "AIoverride"=w150, "type"="Timetrace") -> (w178:T12)
                        n3484 = Reciprocal(x=w165) -> (1/x=w162:dbl)
                        n3485 = local write "refreshtime"(w162) -> ()
                        n3486 = call "2pparameters.vi"("Params in"=w178, "command"="set") -> ()  [unwired: 1 out]
                      }
                      frame "Lifetime (point)" {
                      }
                    }
                  }
                  frame #1 {
                    w183 = FALSE ("wavdet")
                    n3487 = call "2pparameters.vi"("command"="get") -> ("params out"=w187:T12)  [unwired: 1 in]
                    n3488 = Bundle By Name(cluster=w187, "finite"=w183, "cont"=w183, "wavdet"=TRUE) -> (w184:T12)
                    n3489 = call "2pparameters.vi"("Params in"=w184, "command"="set") -> ()  [unwired: 1 out]
                  }
                  frame #2 {
                    n3490 = local read "Meastab"() -> (w214:enum32{"X-Y Image", "Linescan", "Timetrace"})
                    n3491 = property on="AO channels" class="Ring (strict)"() -> ("RingText.Text"=w189:string)  [unwired: 2 in, 2 out]
                    n3492 = property on="refwf" class="Ring (strict)"() -> ("RingText.Text"=w213:string)  [unwired: 2 in, 2 out]
                    n3493 = local read "Build analog waveform tabs"() -> (w212:enum32{"Square", "Triangle", "Matlab"})
                    n3494 = case shown="\"X-Y Image\", Default" w214 {
                      tunnel: [w220 w221] -> w211
                      frame "X-Y Image", Default {
                        n3495 = local read "Sampling rate"() -> (w220:dbl)
                      }
                      frame "Timetrace" {
                        n3496 = local read "srateAODOtt"() -> (w221:dbl)
                      }
                    }
                    n3497 = local read "Matlab waveform path"() -> (w204:path)
                    n3498 = local read "Period (ms)"() -> (w207:dbl)
                    n3499 = local read "Frequency"() -> (w206:dbl)
                    n3500 = local read "Tri Repeats"() -> (w205:dbl)
                    n3501 = local read "Repeats"() -> (w210:dbl)
                    n3502 = local read "Cycles"() -> (w209:dbl)
                    n3503 = local read "Pulses"() -> (w208:dbl)
                    n3504 = call "matlabwfexistsdialogue.vi"("Matlab waveform path"=w204) -> ("mtalab waveform path out"=w203:path)
                    n3505 = call "wfsizecalc.vi"("Sampling frequency (Hz)"=w211, "AOtab"=w212, "reference waveforms to"=w213, "channel"=w189, "Repeats"=w210, "Cycles"=w209, "Matlab wave file"=w203, "pulses"=w208, "Period (ms)"=w207, "Frequency"=w206, "Tri Repeats"=w205) -> ("total size GB"=w198:dbl, "gigabytesize wf"=w194:dbl)  [unwired: 3 in]
                    n3506 = Greater?(x=w194, y=0.5) -> (0:w195:bool)
                    n3507 = Number To Fractional String(number=w194, width (-)=i16 3) -> (F-format string=w200:string)  [unwired: 2 in]
                    n3508 = Number To Fractional String(number=w198, width (-)=i16 4) -> (F-format string=w199:string)  [unwired: 2 in]
                    n3509 = Concatenate Strings("this is a crude approximation:\nyou're about to create a  " ("message"), w200, " GB waveform for a total of " ("string"), w199, " GB. Are you sure?" ("string")) -> (w196:string)
                    n3510 = case shown="True" w195 {
                      tunnel: w196 -> [_ w219]
                      tunnel: [TRUE ("T button?") w216] -> w190
                      frame False {
                      }
                      frame True {
                        n3511 = Two Button Dialog(message=w219, 1:"No, don't do this." ("Center Button Text (\"No\")"), 2:"Yes, continue. " ("Left Button Text (\"Yes\")")) -> (T button?=w216:bool)
                      }
                    }
                  }
                  frame #3 {
                    n3512 = case shown="True" w222 {
                      frame False {
                      }
                      frame True {
                        # "change active waveform numbers array"
                        n3513 = local read "AO channels"() -> (w228:u32)
                        n3514 = call "2pparameters.vi"("command"="get") -> ("params out"=w226:T12)  [unwired: 1 in]
                        n3515 = in-place {
                          in-place-border: w228 -> [w232]
                          in-place-border: [w229] -> w223
                          n3516 = in-place-cluster #49(w226) -> ("aAO"=w231:u32[])
                          n3517 = call "add channel to active arrayv2.vi"("line array in"=w231, "line to add"=w232) -> ("line array out"=w230:u32[], "addition"=w229:bool)  [unwired: 1 out]
                          n3518 = in-place-cluster #49("aAO"=w230) -> (w224:T12)
                        }
                        n3519 = local write "addAO"(w223) -> ()
                        n3520 = call "2pparameters.vi"("Params in"=w224, "command"="set") -> ()  [unwired: 1 out]
                      }
                    }
                  }
                  frame #4 {
                    n3521 = case shown="True" w233 {
                      frame False {
                      }
                      frame True {
                        # "update GUI"
                        n3522 = local read "addAO"() -> (w234:bool)
                        n3523 = case shown="True" w234 {
                          frame False {
                          }
                          frame True {
                            n3524 = call "Used AO lines.vi"() -> ("used AO names"=w238:string[], "used AO lines"=w240:tag[])  [unwired: 2 in]
                            n3525 = control-ref of="Analog Lines Plot"() -> (w239:refnum<vi>)
                            n3526 = control-ref of="Digital Lines Plot"() -> (w237:refnum<vi>)
                            n3527 = call "Used DO lines.vi"() -> ("used DO names"=w236:string[], "used DO lines"=w235:tag[])  [unwired: 2 in]
                            n3528 = local write "Analog Used Lines"(w240) -> ()
                            n3529 = local write "Analog Used Names"(w238) -> ()
                            n3530 = local write "Digital Used Lines"(w235) -> ()
